vi "Configure Arbitrary Waveform Data.vi"(6 "Waveform Generator Number (1: Waveform Generator 1)":i32(ring)=1 items=["Waveform Generator 1"=1, "Waveform Generator 2"=2], 7 "16-bit Integer Data":i32[](array[numeric])=[0], 8 "error in (no error)":errorcluster, 9 "Floating-Point Data":dbl[](array[numeric])=[0.0], 10 "Data Format (0: Floating Point Value)":i32(ring) items=["Floating Point Value", "16-bit Integer Value"], 11 "VISA resource name":refnum<visa-resource-name>) -> (0 "error out":errorcluster, 3 "VISA resource name out":refnum<visa-resource-name>)   [LabVIEW 2016, in "Agilent 2000 3000 X-Series.lvlib"]
doc: "Configures the arbitrary waveform data.\n\n<b>Notes:</b>\n1000 Series do not support this function."
uses:
  Agilent 2000 3000 X-Series.lvlib
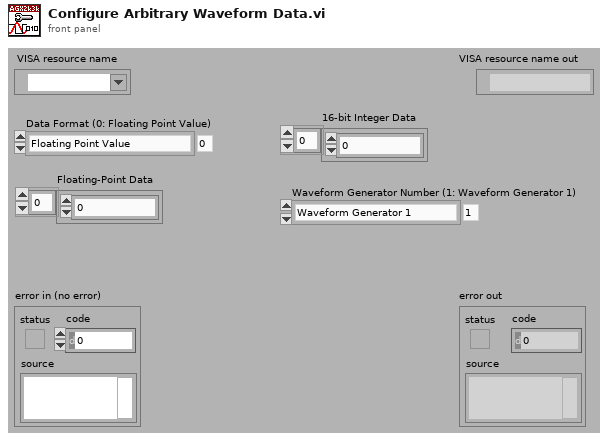
[diagram p1: front panel]
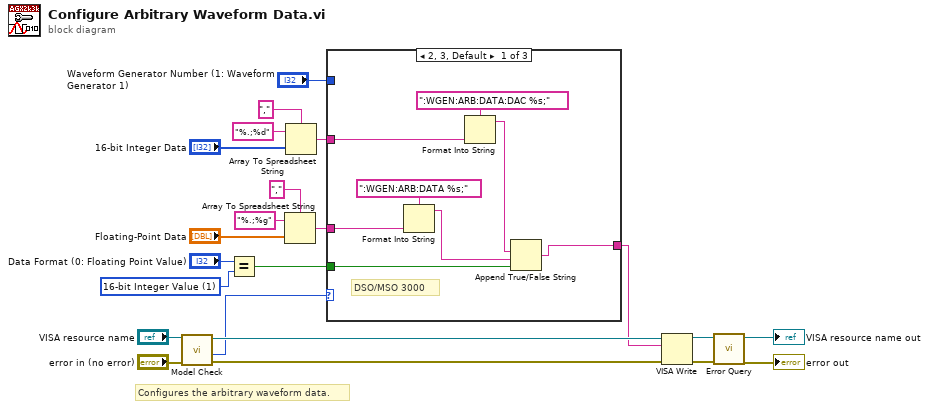
[diagram p0: block diagram]
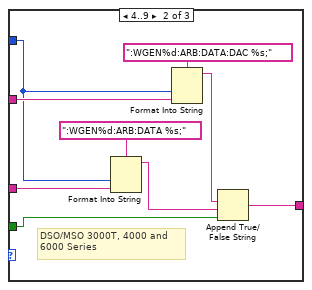
[diagram p2: hidden frame]
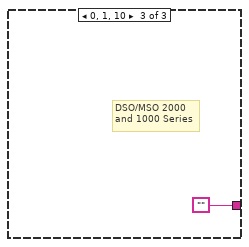
[diagram p3: hidden frame]
diagram:
  w3 = 1 items=["Floating Point Value", "16-bit Integer Value"] ("Data Format (0: Floating Point Value)")
  # "Configures the arbitrary waveform data."
  n1 = call "Model Check.vi"("error in (no error)"="error in (no error)", "VISA resource name"="VISA resource name") -> ("error out"=w11:errorcluster, "Model"=w1:i32, "VISA resource name out"=w12:refnum<visa-resource-name>)  [unwired: 7 out]
  n2 = Equal?(x="Data Format (0: Floating Point Value)", y=w3) -> (x = y?=w2:bool)
  n3 = Array To Spreadsheet String(delimiter (Tab)=",", array="Floating-Point Data", 3:"%.;%g" ("format string")) -> (spreadsheet string=w9:string)
  n4 = Array To Spreadsheet String(delimiter (Tab)=",", array="16-bit Integer Data", 3:"%.;%d" ("format string")) -> (spreadsheet string=w10:string)
  n5 = case shown="2, 3, Default" w1 {
    tunnel: w10 -> [w26 w35 _]
    tunnel: w9 -> [w25 w32 _]
    tunnel: w2 -> [w24 w31 _]
    tunnel: [w23 w34 ""] -> w8
    tunnel: "Waveform Generator Number (1: Waveform Generator 1)" -> [_ w33 _]
    frame 2, 3, Default {
      # "DSO/MSO 3000"
      n6 = Format Into String(format string=":WGEN:ARB:DATA %s;", w25) -> (resulting string=w27:string)  [unwired: 2 in, 1 out]
      n7 = Format Into String(format string=":WGEN:ARB:DATA:DAC %s;", w26) -> (resulting string=w29:string)  [unwired: 2 in, 1 out]
      n8 = Append True/False String(1:w24, 2:w27, 3:w29) -> (0:w23:string)  [unwired: 1 out]
    }
    frame 4..9 {
      # "DSO/MSO 3000T, 4000 and 6000 Series"
      n9 = Format Into String(format string=":WGEN%d:ARB:DATA %s;", w33, w32) -> (resulting string=w36:string)  [unwired: 2 in, 1 out]
      n10 = Format Into String(format string=":WGEN%d:ARB:DATA:DAC %s;", w33, w35) -> (resulting string=w38:string)  [unwired: 2 in, 1 out]
      n11 = Append True/False String(1:w31, 2:w36, 3:w38) -> (0:w34:string)  [unwired: 1 out]
    }
    frame 0, 1, 10 {
      # "DSO/MSO 2000\nand 1000 Series"
    }
  }
  n12 = VISA Write(VISA resource name=w12, write buffer=w8, error in (no error)=w11) -> (VISA resource name out=w22:refnum<visa-resource-name>, error out=w21:errorcluster)  [unwired: 1 out]
  n13 = call "Error Query.vi"("error in (no error)"=w21, "VISA resource name"=w22) -> ("error out"=→"error out":errorcluster, "VISA resource name out"=→"VISA resource name out":refnum<visa-resource-name>)  [unwired: 8 out]
